vi "操作日志写入数据库.vi"(8 "error in (no error)":errorcluster, 11 "data in":T1) -> (0 "error out":errorcluster)   [LabVIEW 2016, in "一代CodMn.lvlib"]
uses:
  <vilib>/Utility/sysdir.llb/System Directory Type.ctl
  <vilib>/addons/database/Connection.llb/DB Tools Open Connec (String).vi
  <vilib>/addons/database/NI_Database_API.lvlib
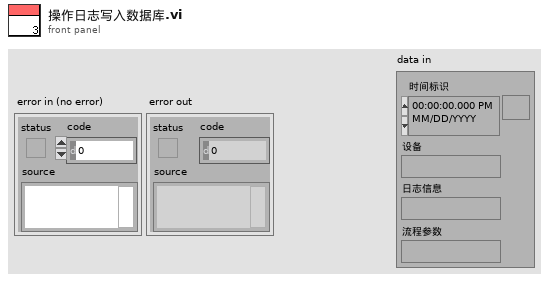
[diagram p1: front panel]
types:
  T1 = cluster{"时间标识":timestamp, "设备":string, "日志信息":string, "流程参数":string}
  T2 = typedef "System Directory Type.ctl" = i32
  T3 = typedef "NI_Database_API.lvlib/Conn ObjectReference.ctl" = refnum<k1>
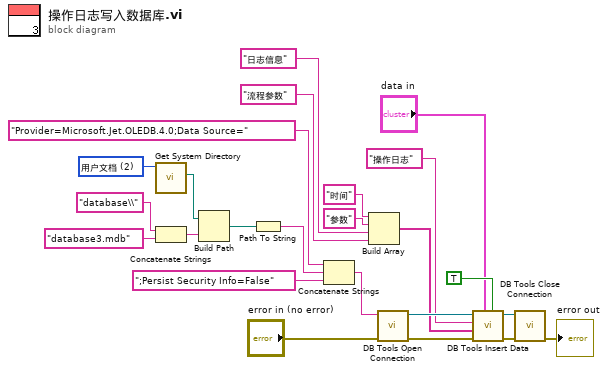
[diagram p0: block diagram]
diagram:
  w17 = T2 2 items=["用户目录"=0, "用户桌面"=1, "用户文档"=2, "用户应用程序数据"=3, "用户设置"=4, "用户临时目录"=5, "公共文档"=6, "公共应用程序数据"=7, "公共设置"=8, "公共缓存"=13, "系统核心库"=9, "系统安装库"=10, "应用程序文件"=11, "启动盘根目录"=12] ("system directory type")
  n1 = call <vilib>:"Get System Directory.vi"("system directory type"=w17) -> ("system directory"=w15:path)  [unwired: 10 in]
  n2 = Concatenate Strings("database\\" ("condition"), "database3.mdb" ("database")) -> (w9:string)
  n3 = Build Path(base path=w15, name or relative path=w9) -> (appended path=w14:path)
  n4 = Path To String(path=w14) -> (string=w13:string)
  n5 = Concatenate Strings("Provider=Microsoft.Jet.OLEDB.4.0;Data Source=" ("condition"), w13, ";Persist Security Info=False" ("condition")) -> (w11:string)
  n6 = Build Array("时间", "参数" ("元素"), "日志信息", "流程参数") -> (w4:string[])
  n7 = call-poly <vilib>:"DB Tools Open Connection.vi"("error in (no error)"="error in (no error)", "connection information"=w11) -> ("error out"=w7:errorcluster, "connection reference"=w8:T3)  [unwired: 6 in]
  n8 = call <vilib>:"DB Tools Insert Data.vi"("create table? (F)"=TRUE, "data"="data in", "error in (no error)"=w7, "columns"=w4, "table"="操作日志", "connection reference"=w8) -> ("error out"=w19:errorcluster, "connection reference out"=w20:T3)  [unwired: 4 in]
  n9 = call <vilib>:"DB Tools Close Connection.vi"("error in (no error)"=w19, "connection reference"=w20) -> ("error out"=→"error out":errorcluster)  [unwired: 5 in]
